vi "dsdll_capture_wave_abort.vi"(8 "error in":errorcluster, 11 "dsdll instance in":T1={"dsdll path"=path "E:/LVprog/DirectSoundDLL/dsdll.dll", "dsdll handle"=[], "output devices"=[], "capture devices"=[]}) -> (0 "error out":errorcluster, 2 "was capturing?":bool, 3 "dsdll instance out":T1)   [LabVIEW 2018, in "dsdll.lvlib"]
doc: "Call this to abort waveform capture. Function is asynchronous so it returns immediately. The 'dsdll instance out' is optional because the function changes nothing in it. So it can be called from a different thread/process."
uses:
  dsdll.lvlib
  dsdll_instance.ctl
  dsdll_device_record.ctl
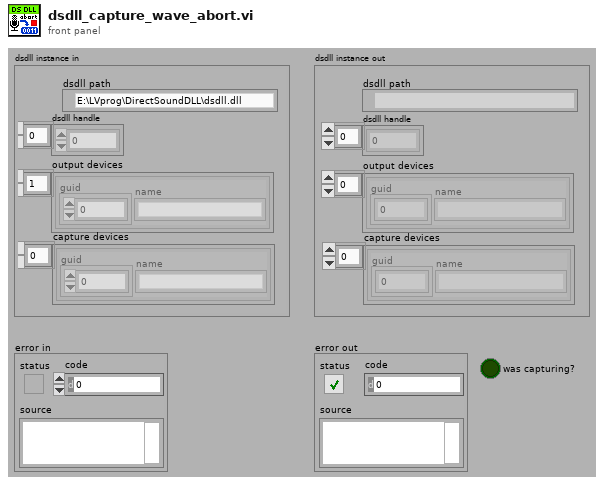
[diagram p1: front panel]
types:
  T1 = typedef "dsdll.lvlib/dsdll_instance.ctl" = cluster{"dsdll path":path, "dsdll handle":u8[], "output devices":T2[], "capture devices":T2[]}
  T2 = typedef "dsdll.lvlib/dsdll_device_record.ctl" = cluster{"guid":u8[], "name":string}
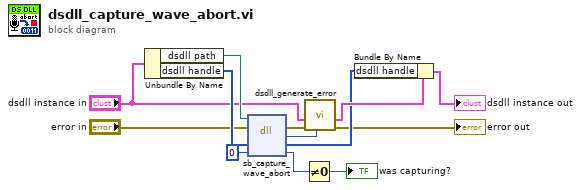
[diagram p0: block diagram]
diagram:
  n1 = Unbundle By Name("dsdll instance in") -> ("dsdll path"=w9:path, "dsdll handle"=w8:u8[])
  n2 = dll-call lib="dsdll.dll" fn="sb_capture_wave_abort" ("sb_get_handle_size()")(path in=w9, error in="error in", "handle"=w8, "was_runnig"=0) -> (error out=w13:errorcluster, "error"=w12:i32, "handle"=w10:u8[], "was_runnig"=w2:i32)  [unwired: 1 in, 1 out]
  n3 = Not Equal To 0?(x=w2) -> (x != 0?=→"was capturing?":bool)
  n4 = call "dsdll_generate_error.vi"("error code"=w12, "error in"=w13, "dsdll instance in"="dsdll instance in") -> ("error out"=→"error out":errorcluster, "dsdll instance out"=w11:T1)  [unwired: 6 in, 1 out]
  n5 = Bundle By Name(cluster=w11, "dsdll handle"=w10) -> (→"dsdll instance out":T1)
